vi "ForceWait.vi"() -> ()   [LabVIEW 2012]
panel:
  in  "ForceWait":bool
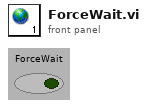
[diagram p1: front panel]
diagram:
